vi "ControlArmInterface.vi"() -> ()   [LabVIEW 2024]
uses:
  <vilib>/Instr/_visa.llb/VISA Configure Serial Port (Instr).vi
panel:
  in  "baud rate (9600)":u32=9600
  out "string 2":string
  out "concatenated string":string
  out "string":string
  in  "Power Button":bool
  in  "Position Maximum":bool
  in  "Position Minimum":bool
  in  "BackwardButton":bool
  in  "ForwardButton":bool
  in  "ScramButton":bool
  in  "SpeedSelectButton":bool
  in  "ElectormagnetButton":bool
  out "Analog In 4":u16(slide)=187 scale=0.0..1023.0
  out "Analog In 3":u16(slide)=187 scale=0.0..1023.0
  out "Analog In 2":u16(slide)=187 scale=0.0..1023.0
  out "Analog In 1":u16(knob)=187 scale=0.0..1023.0
  out "Digital Inputs 2":bool[](array[boolean])=[TRUE, TRUE, TRUE, TRUE, TRUE, TRUE, TRUE, TRUE]
  out "Digital Inputs":bool[](array[boolean])=[TRUE, TRUE, TRUE, TRUE, TRUE, TRUE, TRUE, TRUE]
  out "Hex data received":string
  in  "stop":bool
  in  "VISA resource name":refnum<visa-resource-name>
  # "Analog Inputs"
  # "Digital Indicators"
  # "Debug Section"
  # "Motor Active"
  # "Scram Bit\nPower Bit\nMagnet Bit\nForward Bit\nBackward Bit\nMinimum Position \nMaximum Position\nSpeed Select Bit"
  # "Digital Buttons"
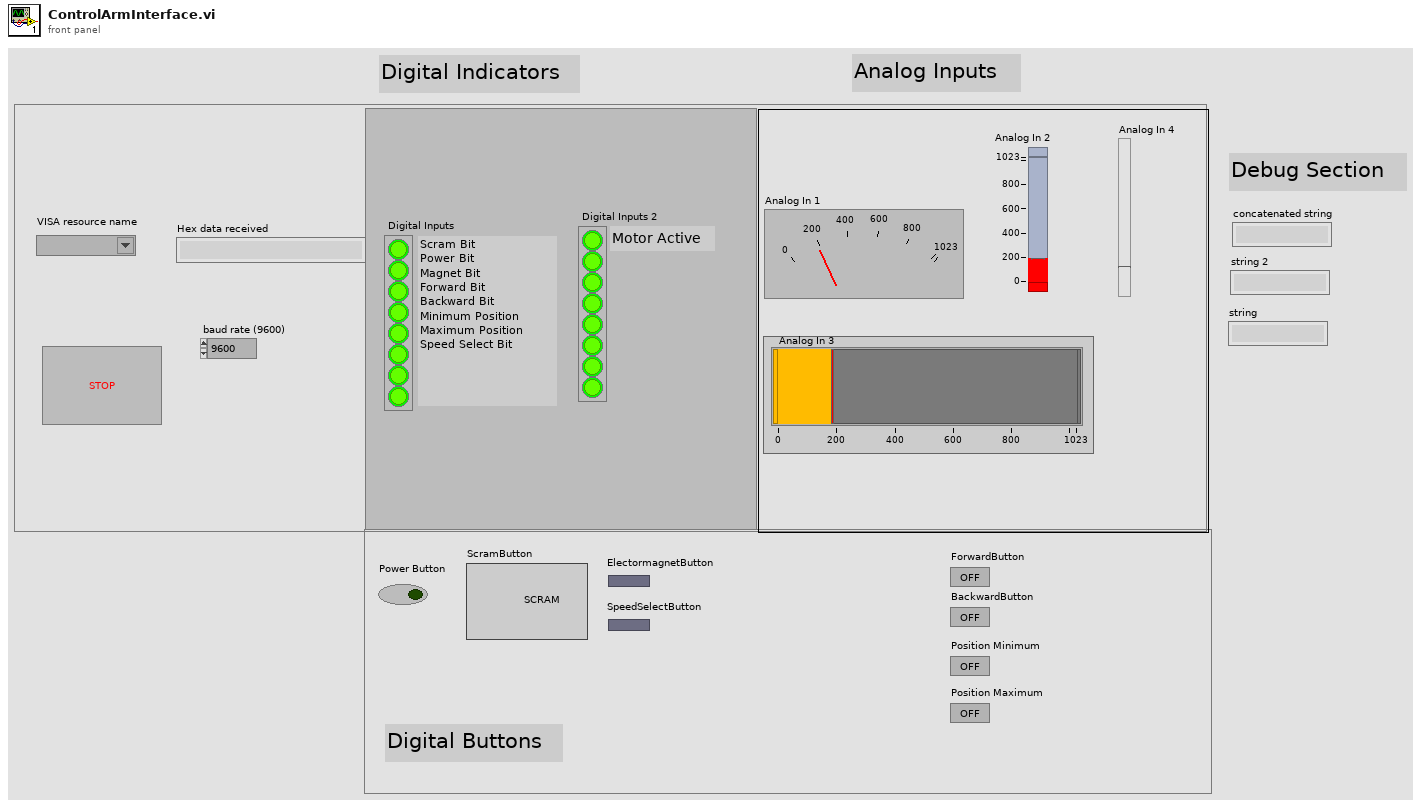
[diagram p1: front panel]
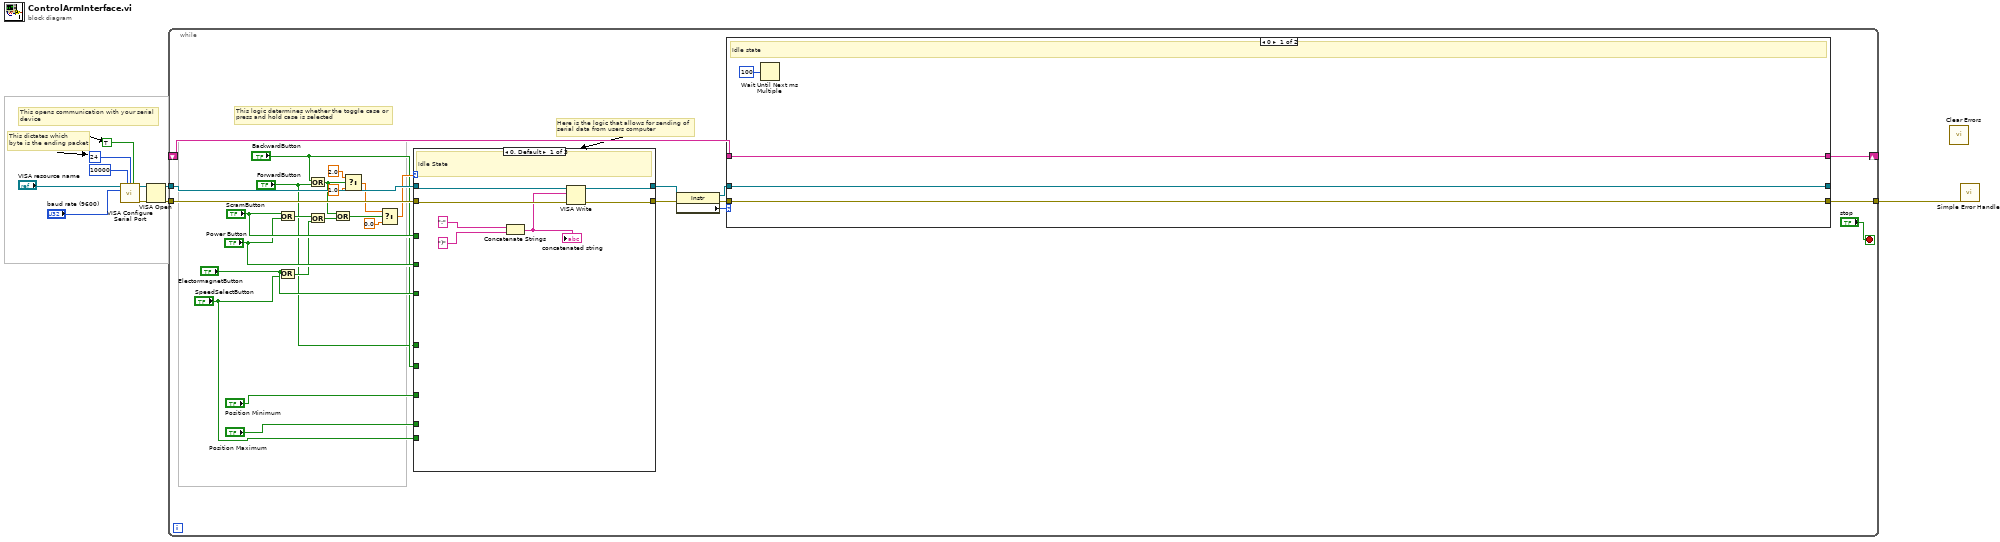
[diagram p0: block diagram]
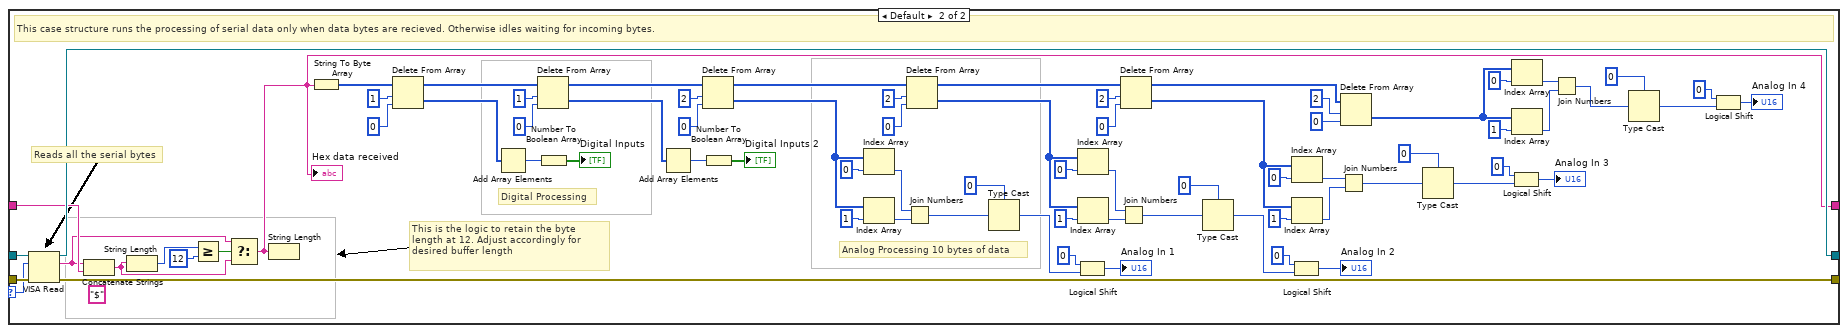
[diagram p2: hidden frame]
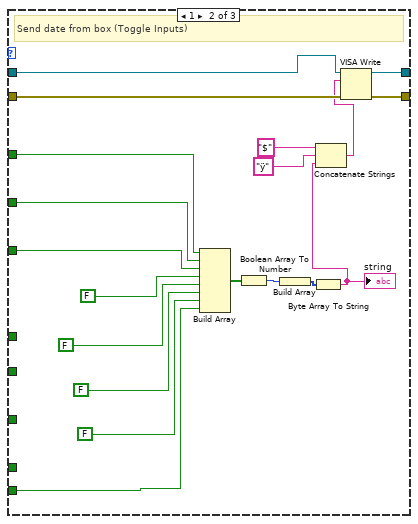
[diagram p3: hidden frame]
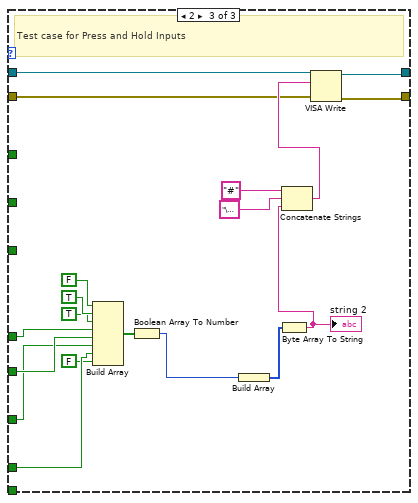
[diagram p4: hidden frame]
diagram:
  # "This dictates which\nbyte is the ending packet"
  # "This opens communication with your serial\ndevice"
  n1 = call-poly "VISA Configure Serial Port"("VISA resource name"="VISA resource name", "timeout (10sec)"=u32 10000, "termination char\n(0xA = '\\n' = LF)"=u8 24 ("termination char\n(0xA = '\\n' = LF)"), "Enable Termination\nChar (T)"=TRUE ("Enable Termination\nChar (T)"), "baud rate (9600)"="baud rate (9600)") -> ("VISA resource name out"=w6:refnum<visa-resource-name>, "error out"=w5:errorcluster)  [unwired: 9 in]
  n2 = VISA Open(error in (no error)=w5, VISA resource name=w6) -> (VISA resource name=w4:refnum<visa-resource-name>, error out=w3:errorcluster)  [unwired: 3 in]
  n3 = while {
    shift-right: [w33] -> _
    shift-left: _ -> [w32]
    tunnel: w4 -> [w31]
    tunnel: w3 -> [w30]
    tunnel: [w29] -> w2
    stop <- "stop" stop-if-true
    # "This logic determines whether the toggle case or \npress and hold case is selected"
    # "Here is the logic that allows for sending of \nserial data from users computer"
    n4 = Or(x="ScramButton", y="Power Button") -> (x .or. y?=w23:bool)
    n5 = Or(x="ElectormagnetButton", y="SpeedSelectButton") -> (x .or. y?=w24:bool)
    n6 = Or(x="BackwardButton", y="ForwardButton") -> (x .or. y?=w13:bool)
    n7 = Or(x=w23, y=w24) -> (x .or. y?=w14:bool)
    n8 = Or(x=w13, y=w14) -> (x .or. y?=w12:bool)
    n9 = Select(t=2.0, s=w13, f=1.0) -> (s? t:f=w22:dbl)
    n10 = Select(t=w22, s=w12, f=0.0) -> (s? t:f=w21:dbl)
    n11 = case shown="0, Default" w21 {
      tunnel: [w125 w145 w156] -> w37
      tunnel: w31 -> [w124 w144 w155]
      tunnel: w30 -> [w123 w143 w154]
      tunnel: [w126 w142 w157] -> w38
      tunnel: "Power Button" -> [_ w138 _]
      tunnel: "ScramButton" -> [_ w137 _]
      tunnel: "SpeedSelectButton" -> [_ w131 _]
      tunnel: "ElectormagnetButton" -> [_ w136 _]
      tunnel: "ForwardButton" -> [_ _ w150]
      tunnel: "BackwardButton" -> [_ _ w149]
      tunnel: "Position Minimum" -> [_ _ w148]
      tunnel: "Position Maximum" -> [_ _ w147]
      frame 0, Default {
        # "Idle State"
        n12 = Concatenate Strings(":", ")") -> (w120:string)
        "concatenated string" <- w120
        n13 = VISA Write(VISA resource name=w124, write buffer=w120, error in (no error)=w123) -> (VISA resource name out=w126:refnum<visa-resource-name>, error out=w125:errorcluster)  [unwired: 1 out]
      }
      frame 1 {
        # "Send date from box (Toggle Inputs)"
        n14 = Build Array(w137, w138, w136, FALSE ("ForwardButton"), FALSE ("BackwardButton"), FALSE ("Position Minimum"), FALSE ("Position Maximum"), w131) -> (w139:bool[])
        n15 = Boolean Array To Number(Boolean array=w139) -> (number=w140:u32)
        n16 = Build Array(w140) -> (w141:u32[])
        n17 = Byte Array To String(unsigned byte array=w141) -> (string=w132:string)
        "string" <- w132
        n18 = Concatenate Strings "Concatenate Strings"("$" ("element"), "ÿ" ("string"), w132) -> (w135:string)
        n19 = VISA Write(VISA resource name=w144, write buffer=w135, error in (no error)=w143) -> (VISA resource name out=w142:refnum<visa-resource-name>, error out=w145:errorcluster)  [unwired: 1 out]
      }
      frame 2 {
        # "Test case for Press and Hold Inputs"
        n20 = Build Array "Build Array"(FALSE, TRUE, TRUE, w150, w149, w148, w147, FALSE) -> (w162:bool[])
        n21 = Boolean Array To Number(Boolean array=w162) -> (number=w163:u32)
        n22 = Build Array "Build Array"(w163) -> (w164:u32[])
        n23 = Byte Array To String(unsigned byte array=w164) -> (string=w158:string)
        "string 2" <- w158
        n24 = Concatenate Strings "Concatenate Strings"("#" ("element"), "\u0000" ("string"), w158) -> (w161:string)
        n25 = VISA Write(VISA resource name=w155, write buffer=w161, error in (no error)=w154) -> (VISA resource name out=w157:refnum<visa-resource-name>, error out=w156:errorcluster)  [unwired: 1 out]
      }
    }
    n26 = property class="Instr"(reference=w38, error in=w37) -> (reference out=w36:refnum<visa-resource-name>, error out=w35:errorcluster, "Serial Settings:Number of Bytes at Serial Port"=w34:u32)
    n27 = case shown="0" w34 {
      selector: w34 -> [_ w115]
      tunnel: [w43 w119] -> _
      tunnel: [w42 w118] -> w29
      tunnel: w36 -> [w43 w117]
      tunnel: w35 -> [w42 w116]
      tunnel: w32 -> [w40 w114]
      tunnel: [w40 w102] -> w33
      frame 0 {
        # "Idle state"
        n28 = Wait Until Next ms Multiple(millisecond multiple=u32 100 ("millisecond timer value")) -> ()  [unwired: 1 out]
      }
      frame Default {
        (unwired) "$"
        # "Analog Processing 10 bytes of data"
        # "Digital Processing"
        # "This is the logic to retain the byte length at 12. Adjust accordingly for \ndesired buffer length"
        # "Reads all the serial bytes"
        # "This case structure runs the processing of serial data only when data bytes are recieved. Otherwise idles waiting for incoming bytes."
        n29 = VISA Read(VISA resource name=w117, byte count=w115, error in (no error)=w116) -> (VISA resource name out=w119:refnum<visa-resource-name>, read buffer=w110:string, error out=w118:errorcluster)  [unwired: 1 out]
        n30 = Concatenate Strings(w110, w114) -> (w109:string)
        n31 = String Length(string=w109) -> (length=w113:i32)
        n32 = Greater Or Equal?(x=w113, y=12) -> (x >= y?=w111:bool)
        n33 = Select(t=w110, s=w111, f=w109) -> (s? t:f=w102:string)
        "Hex data received" <- w102
        n34 = String Length(string=w102) -> ()  [unwired: 1 out]
        n35 = String To Byte Array(string=w102) -> (unsigned byte array=w107:u8[])
        n36 = Delete From Array "Delete From Array"(array=w107, length=1, index=0) -> (deleted portion=w108:u8[], array with subset deleted=w98:u8[])
        n37 = Add Array Elements(numeric array=w108) -> (sum=w106:u8)
        n38 = Delete From Array "Delete From Array"(array=w98, length=1, index=0) -> (deleted portion=w99:u8[], array with subset deleted=w48:u8[])
        n39 = Number To Boolean Array(number=w106) -> (Boolean array=→"Digital Inputs":bool[])
        n40 = Add Array Elements(numeric array=w99) -> (sum=w96:u8)
        n41 = Delete From Array "Delete From Array"(array=w48, length=2, index=0) -> (deleted portion=w89:u8[], array with subset deleted=w47:u8[])
        n42 = Number To Boolean Array(number=w96) -> (Boolean array=→"Digital Inputs 2":bool[])
        n43 = Index Array(array=w89, index=0) -> (element=w86:u8)
        n44 = Index Array(array=w89, index=1) -> (element=w85:u8)
        n45 = Join Numbers(hi=w86, lo=w85) -> ((hi.lo)=w84:u16)
        n46 = Delete From Array "Delete From Array"(array=w47, length=2, index=0) -> (deleted portion=w78:u8[], array with subset deleted=w46:u8[])
        n47 = Type Cast(type=u16 0 ("y"), x=w84) -> (*(type *) &x=w93:u16)
        n48 = Logical Shift(y=i16 0, x=w93) -> (x << y=→"Analog In 1":u16)
        n49 = Index Array(array=w78, index=0) -> (element=w81:u8)
        n50 = Index Array(array=w78, index=1) -> (element=w82:u8)
        n51 = Join Numbers(hi=w81, lo=w82) -> ((hi.lo)=w83:u16)
        n52 = Delete From Array "Delete From Array"(array=w46, length=2, index=0) -> (deleted portion=w65:u8[], array with subset deleted=w45:u8[])
        n53 = Type Cast(type=u16 0 ("y"), x=w83) -> (*(type *) &x=w74:u16)
        n54 = Logical Shift(y=i16 0, x=w74) -> (x << y=→"Analog In 2":u16)
        n55 = Index Array(array=w65, index=0) -> (element=w62:u8)
        n56 = Index Array(array=w65, index=1) -> (element=w61:u8)
        n57 = Join Numbers(hi=w62, lo=w61) -> ((hi.lo)=w60:u16)
        n58 = Delete From Array "Delete From Array"(array=w45, length=2, index=0) -> (deleted portion=w55:u8[])  [unwired: 1 out]
        n59 = Type Cast(type=u16 0 ("y"), x=w60) -> (*(type *) &x=w69:u16)
        n60 = Logical Shift(y=i16 0, x=w69) -> (x << y=→"Analog In 3":u16)
        n61 = Index Array(array=w55, index=0) -> (element=w57:u8)
        n62 = Index Array(array=w55, index=1) -> (element=w58:u8)
        n63 = Join Numbers(hi=w57, lo=w58) -> ((hi.lo)=w59:u16)
        n64 = Type Cast(type=u16 0 ("y"), x=w59) -> (*(type *) &x=w51:u16)
        n65 = Logical Shift(y=i16 0, x=w51) -> (x << y=→"Analog In 4":u16)
      }
    }
  }
  n66 = call <vilib>:"Clear Errors.vi"() -> ()  [unwired: 6 in, 2 out]
  n67 = call <vilib>:"Simple Error Handler.vi"("error in (no error)"=w2) -> ()  [unwired: 4 in, 5 out]
